vi "SensorConsole.vi"(8 "error in (no error)":errorcluster) -> (0 "error out":errorcluster)   [LabVIEW 2013, in "SensorConsoleLib.lvlib"]
doc: "This Console provides access to Funds dispensed and Received."
uses:
  SensorConsoleLib.lvlib
  PrivateControls/SensorConsole_QueueDriver.ctl
  MainVI/TopLevelController/ToplevelControllerLibrary.lvlib
  UserConsole/UserConsole.lvlib
panel:
  in  "Funds":bool
  in  "Deposit":bool
  # "This Console provides access to Funds dispensed and Received."
  # "[Covers: UI1]"
  # "[Covers: UI4] \n[Covers: UI4A] \n[Covers: UI4B]"
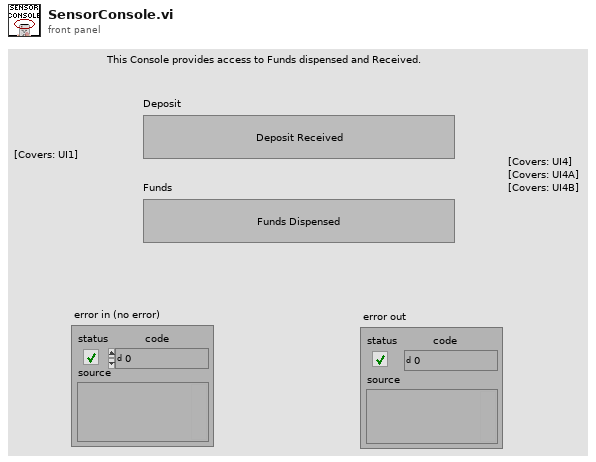
[diagram p1: front panel]
types:
  T1 = typedef "SensorConsoleLib.lvlib/SensorConsole_QueueDriver.ctl" = enum16{"Default case", "Init", "Enqueue", "Dequeue", "ReleaseQueue", "Exit"}
  T2 = enum16{"Create Event", "Generate Event", "Destroy Event"}
  T3 = enum16{"Init", "Enqueue", "Dequeue", "ReleaseQueue", "Exit"}
  T4 = typedef "SensorConsoleLib.lvlib/DataCluster_SensorConsole.ctl" = cluster{"Deposit":bool, "Funds":bool}
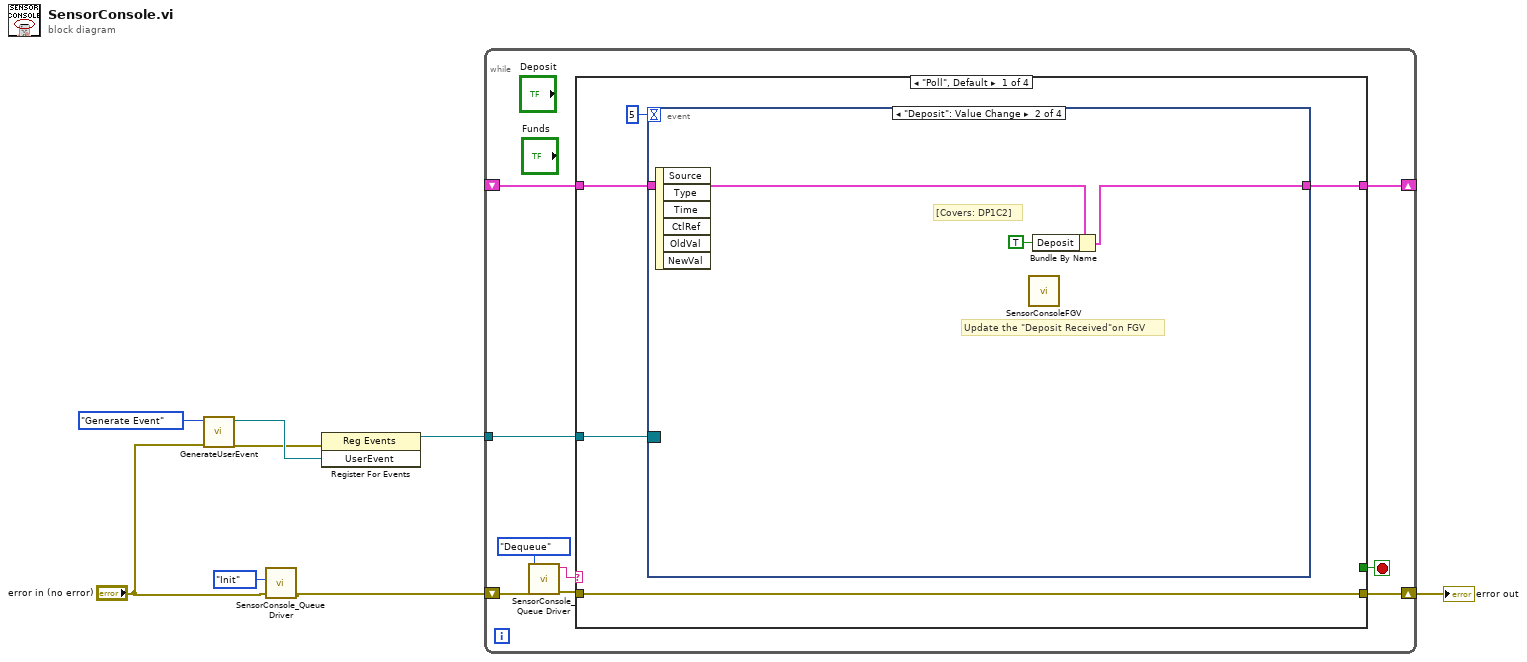
[diagram p0: block diagram]
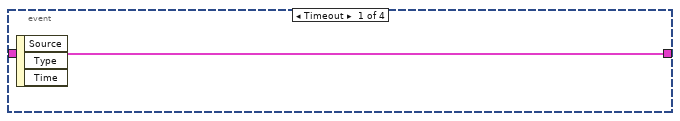
[diagram p2: hidden frame]
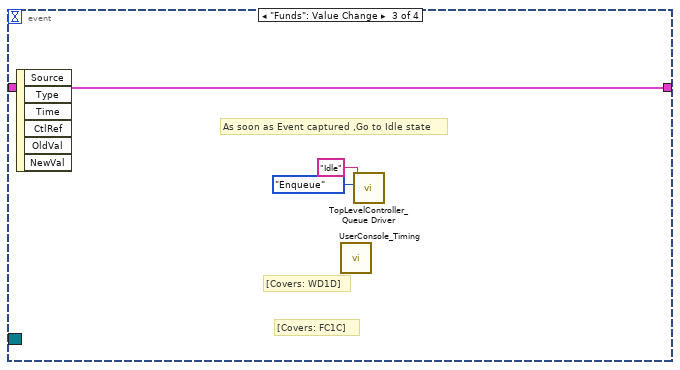
[diagram p3: hidden frame]
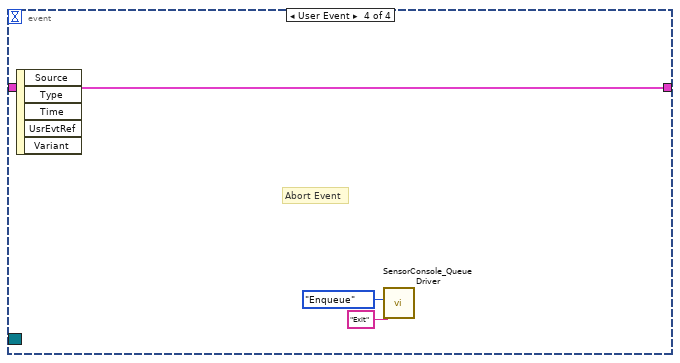
[diagram p4: hidden frame]
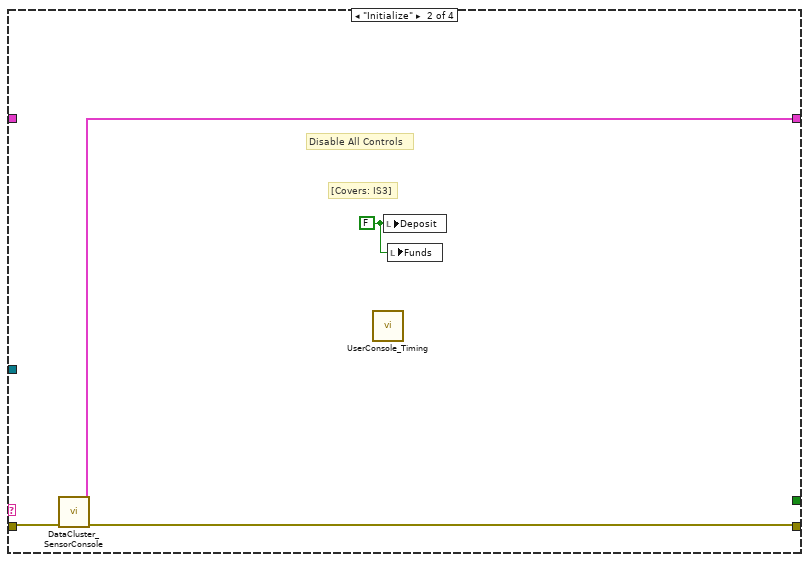
[diagram p5: hidden frame]
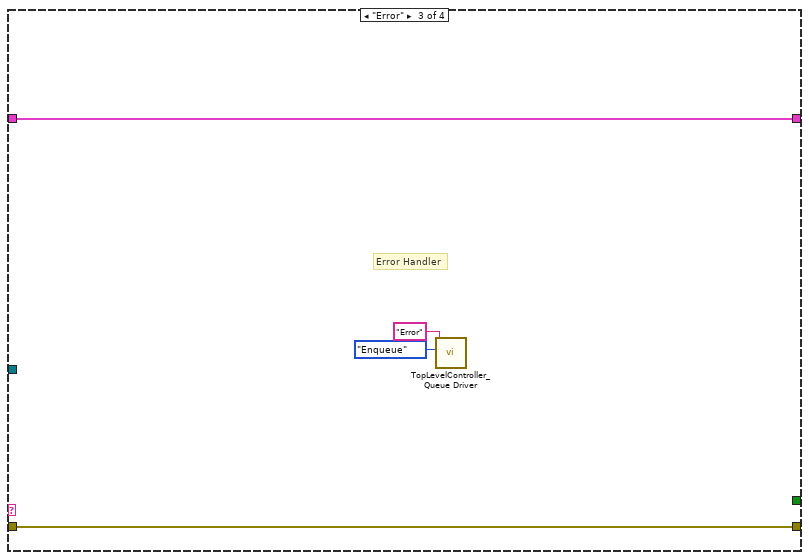
[diagram p6: hidden frame]
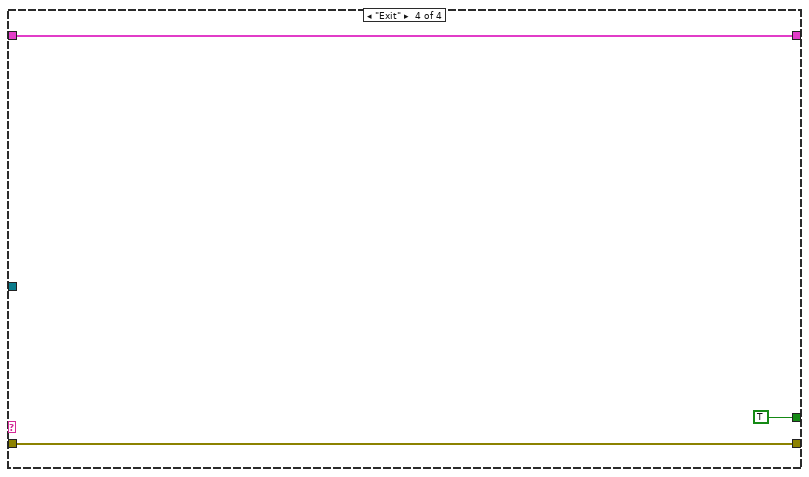
[diagram p7: hidden frame]
diagram:
  n1 = call "GenerateUserEvent.vi"("error in (no error)"="error in (no error)", "Event Actions"=T2."Generate Event") -> ("error out"=w4:errorcluster, "UserEvent"=w5:refnum<user-event>)  [unwired: 8 in]
  n2 = call "SensorConsole_Queue Driver.vi"("error in (no error)"="error in (no error)", "Enum"=SensorConsole_QueueDriver."Init") -> ("error out"=w7:errorcluster)  [unwired: 8 in, 1 out]
  n3 = register-events(error in=w4, w5) -> (reference out=w3:refnum<event-registration>)  [unwired: 1 in, 1 out]
  n4 = while {
    shift-right: [w16] -> _
    shift-left: _ -> [w15]
    shift-right: [w17] -> w8
    shift-left: w7 -> [w12]
    tunnel: w3 -> [w10]
    stop <- w11 stop-if-true
    n5 = call "SensorConsole_Queue Driver.vi"("error in (no error)"=w12, "Enum"=SensorConsole_QueueDriver."Dequeue") -> ("error out"=w14:errorcluster, "DeQ"=w13:string)  [unwired: 8 in]
    n6 = case shown="\"Poll\", Default" w13 {
      tunnel: w14 -> [w22 w36 w39 w43]
      tunnel: [w22 w34 w39 w43] -> w17
      tunnel: [w20 w35 w40 w41] -> w16
      tunnel: w15 -> [w21 _ w40 w41]
      tunnel: [_ _ _ TRUE] -> w11
      tunnel: w10 -> [w19 _ _ _]
      frame "Poll", Default {
        n7 = event shown="[1] \"Deposit\": Value Change" {
          selector: w19 -> [_ _ _ _]
          dyn-events: _ -> [_ _ _ _]
          timeout: 5 -> [_ _ _ _]
          tunnel: w21 -> [w23 w26 w29 w31]
          tunnel: [w23 w25 w29 w31] -> w20
          event Timeout {
            n8 = event-data() -> ()  [unwired: 1 in, 3 out]
          }
          event "Deposit": Value Change {
            # "[Covers: DP1C2]"
            # "Update the \"Deposit Received\"on FGV"
            n9 = event-data() -> ()  [unwired: 1 in, 6 out]
            n10 = call "SensorConsoleFGV.vi"() -> ()  [unwired: 10 in, 2 out]
            n11 = Bundle By Name(cluster=w26, "Deposit"=TRUE) -> (w25:T4)
          }
          event "Funds": Value Change {
            # "[Covers: FC1C]"
            # "[Covers: WD1D]"
            # "As soon as Event captured ,Go to Idle state"
            n12 = event-data() -> ()  [unwired: 1 in, 6 out]
            n13 = call "UserConsole_Timing.vi"() -> ()  [unwired: 11 in, 1 out]
            n14 = call "TopLevelController_Queue Driver.vi"("Enum"=T3."Enqueue", "EnQ"="Idle") -> ()  [unwired: 8 in, 2 out]
          }
          event User Event {
            # "Abort Event"
            n15 = event-data() -> ()  [unwired: 1 in, 5 out]
            n16 = call "SensorConsole_Queue Driver.vi"("Enum"=SensorConsole_QueueDriver."Enqueue", "EnQ"="Exit") -> ()  [unwired: 8 in, 2 out]
          }
        }
      }
      frame "Initialize" {
        w33 = FALSE ("Deposit")
        # "[Covers: IS3]"
        # "Disable All Controls"
        n17 = call "DataCluster_SensorConsole.vi"("error in (no error)"=w36) -> ("error out"=w34:errorcluster, "Data Cluster"=w35:T4)  [unwired: 9 in]
        n18 = call "UserConsole_Timing.vi"() -> ()  [unwired: 11 in, 1 out]
        n19 = local write "Deposit"(w33) -> ()
        n20 = local write "Funds"(w33) -> ()
      }
      frame "Error" {
        # "Error Handler"
        n21 = call "TopLevelController_Queue Driver.vi"("Enum"=T3."Enqueue", "EnQ"="Error") -> ()  [unwired: 8 in, 2 out]
      }
      frame "Exit" {
      }
    }
  }
  "error out" <- w8
